vi "interchannel delay.vi"(5 "Server Method":T1={"scan rate (Hz)"=100.0, "Channel group array"=[], "Number of groups"=1} {"Number of groups" min=1; "Channel group array"."max voltage" format="%.4f"; "scan rate (Hz)" format="%.2f"}) -> (2 "interchannel delay\nin secs ( -1: hw default)":sgl=-1.0 format="%^.2e")   [LabVIEW 2010]
uses:
  Dataserver method.ctl
panel:
  # "Hz"
  # "channel identifiers"
  # "max voltage"
  # "port locations"
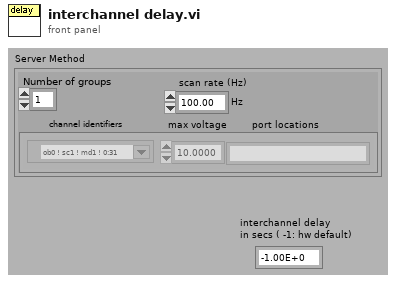
[diagram p1: front panel]
types:
  T1 = typedef "Dataserver method.ctl" = cluster{"scan rate (Hz)":dbl, "Channel group array":cluster{"channels":tag, "max voltage":sgl, "Port locations":string}[], "Number of groups":u8}
  T2 = cluster{"channels":tag, "max voltage":sgl, "Port locations":string}[]
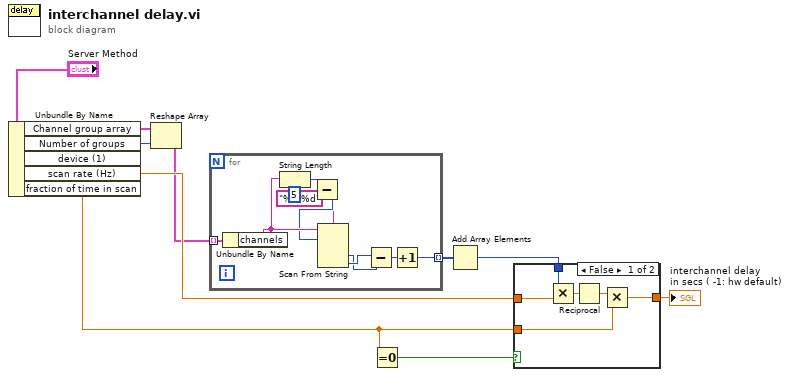
[diagram p0: block diagram]
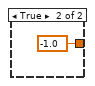
[diagram p2: hidden frame]
diagram:
  n1 = Unbundle By Name("Server Method") -> ("Channel group array"=w4:T2, "Number of groups"=w5:u8, "scan rate (Hz)"=w9:dbl, "fraction of time in scan"=w7:dbl)  [unwired: 1 out]
  n2 = Reshape Array(w4, w5) -> (w3:T2)
  n3 = for {
    tunnel: w3 -> [w20] mode=indexing
    tunnel: [w11] -> w2 mode=indexing
    n4 = Unbundle By Name(w20) -> ("channels"=w19:tag)
    n5 = String Length(string=w19) -> (length=w18:i32)
    n6 = Subtract(x=w18, y=5) -> (x-y=w16:i32)
    n7 = Scan From String(format string="%d:%d", input string=w19, initial scan location=w16) -> (output 1=w13:i32, output 2=w14:i32)  [unwired: 3 in, 3 out]
    n8 = Subtract(x=w14, y=w13) -> (x-y=w12:i32)
    n9 = Increment(x=w12) -> (x+1=w11:i32)
  }
  n10 = Equal To 0?(x=w7) -> (x = 0?=w6:bool)
  n11 = Add Array Elements(numeric array=w2) -> (sum=w1:i32)
  n12 = case shown="False" w6 {
    tunnel: w1 -> [w26 _]
    tunnel: w9 -> [w25 _]
    tunnel: [w22 -1.0] -> w8
    tunnel: w7 -> [w21 _]
    frame False {
      n13 = Multiply(x=w26, y=w25) -> (x*y=w24:dbl)
      n14 = Reciprocal(x=w24) -> (1/x=w23:dbl)
      n15 = Multiply(x=w23, y=w21) -> (x*y=w22:dbl)
    }
    frame True {
    }
  }
  "interchannel delay\nin secs ( -1: hw default)" <- w8
